vi "Close.vi"(8 "error in (no error)":errorcluster) -> (0 "error out":errorcluster)   [LabVIEW 2020, in "输出轴伺服.lvlib"]
uses:
  Servo_global.vi
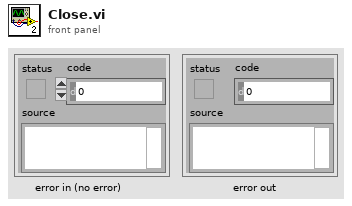
[diagram p1: front panel]
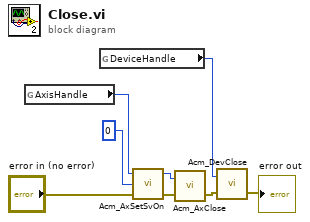
[diagram p0: block diagram]
diagram:
  n1 = global read "Servo_global.vi" "AxisHandle"() -> (w3:u32)
  n2 = global read "Servo_global.vi" "DeviceHandle"() -> (w6:u32)
  n3 = call <userlib>:"Acm_AxSetSvOn.vi"("Error Input(No Error)"="error in (no error)", "OnOff"=u32 0, "AxisHandle"=w3) -> ("Error Output"=w1:errorcluster, "AxisHandle"=w2:u32)  [unwired: 1 out]
  n4 = call <userlib>:"Acm_AxClose.vi"("Error Input(No Error)"=w1, "AxisHandle"=w2) -> ("Error Output"=w8:errorcluster)  [unwired: 1 out]
  n5 = call <userlib>:"Acm_DevClose.vi"("Error Input(No Error)"=w8, "DeviceHandle"=w6) -> ("Error Output"=→"error out":errorcluster)  [unwired: 1 out]
